vi "Initialize.vi"(0 "CS in":refnum<class "CS.lvclass">, 5 "HW Address":u32, 11 "error in (no error)":errorcluster) -> (4 "CS out":refnum<class "CS.lvclass">, 6 "Instrument ID":string, 15 "error out":errorcluster)   [LabVIEW 2016, in "CS.lvclass"]
uses:
  Lib.llb/CS.lvclass
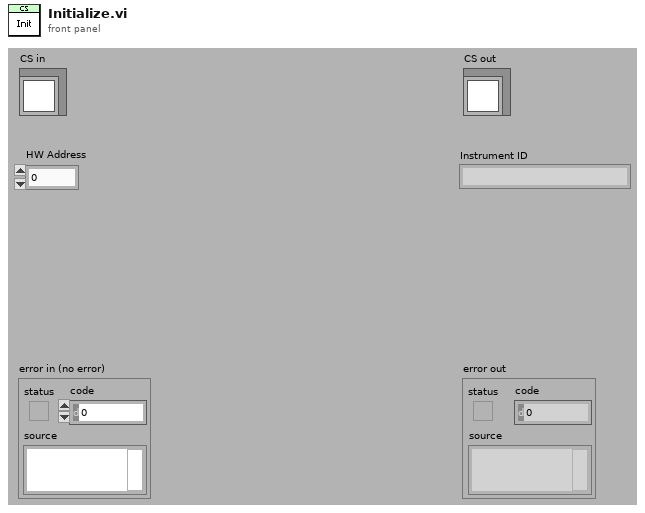
[diagram p1: front panel]
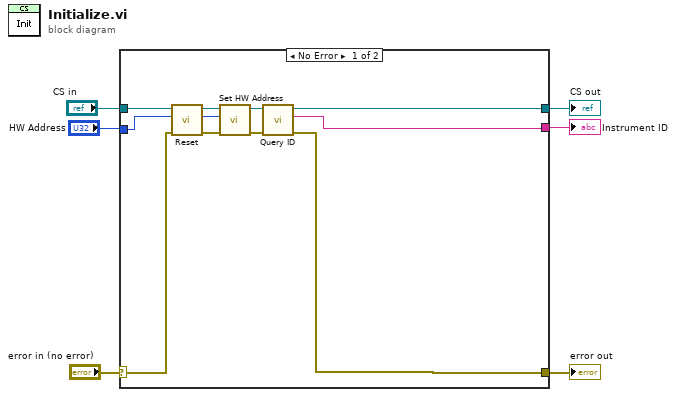
[diagram p0: block diagram]
diagram:
  n1 = case shown="No Error" "error in (no error)" {
    selector: "error in (no error)" -> [w12 w18]
    tunnel: [w15 w18] -> w5
    tunnel: [w14 w17] -> w3
    tunnel: "CS in" -> [w11 w17]
    tunnel: "HW Address" -> [w16 _]
    tunnel: [w13 _] -> w1
    frame No Error {
      n2 = call-dynamic "Reset.vi"("error in (no error)"=w12, "CS in"=w11) -> ("error out"=w9:errorcluster, "CS out"=w10:refnum<class "CS.lvclass">)  [unwired: 8 in]
      n3 = call-dynamic "Set HW Address.vi"("error in (no error)"=w9, "HW Address"=w16, "CS.lvclass in"=w10) -> ("error out"=w7:errorcluster, "CS.lvclass out"=w8:refnum<class "CS.lvclass">)  [unwired: 7 in]
      n4 = call-dynamic "Query ID.vi"("error in (no error)"=w7, "DMM in"=w8) -> ("error out"=w15:errorcluster, "ID  string"=w13:string, "DMM out"=w14:refnum<class "CS.lvclass">)  [unwired: 7 in]
    }
    frame Error {
    }
  }
  "error out" <- w5
  "CS out" <- w3
  "Instrument ID" <- w1
